vi "Agilent B2900 Series Output DC Volts.vi"() -> ()   [LabVIEW 2023]
doc: "This example shows how to configure the instrument's output voltage level, over current protection, and over voltage protection. The actual voltage level and actual current level are returned as well as whether over voltage protection (OVP) or over current protection (OCP) has been tripped."
uses:
  Agilent B2900 Series.lvlib
panel:
  in  "Source Range (V)":dbl=2.0
  in  "Voltage Level (V)":dbl
  in  "Compliance Current (0.0001 A)":dbl=0.0001
  in  "Enable Output Protection (T: Enable)":bool=TRUE
  in  "Stop Output":bool
  out "OCP Tripped?":bool
  out "Actual Current Level (A)":dbl format="%_6g"
  out "Actual Voltage Level (V)":dbl format="%_6g"
  in  "Channel (0: Channel 1)":i32(ring) items=["Channel 1", "Channel 2"]
  in  "VISA resource name":refnum<visa-resource-name>
  # "(c) 2011-2021 National Instruments.  ALL RIGHTS RESERVED."
  # "Compliance Protection"
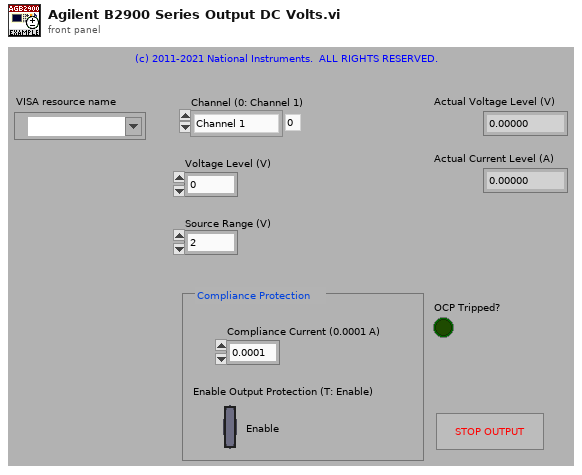
[diagram p1: front panel]
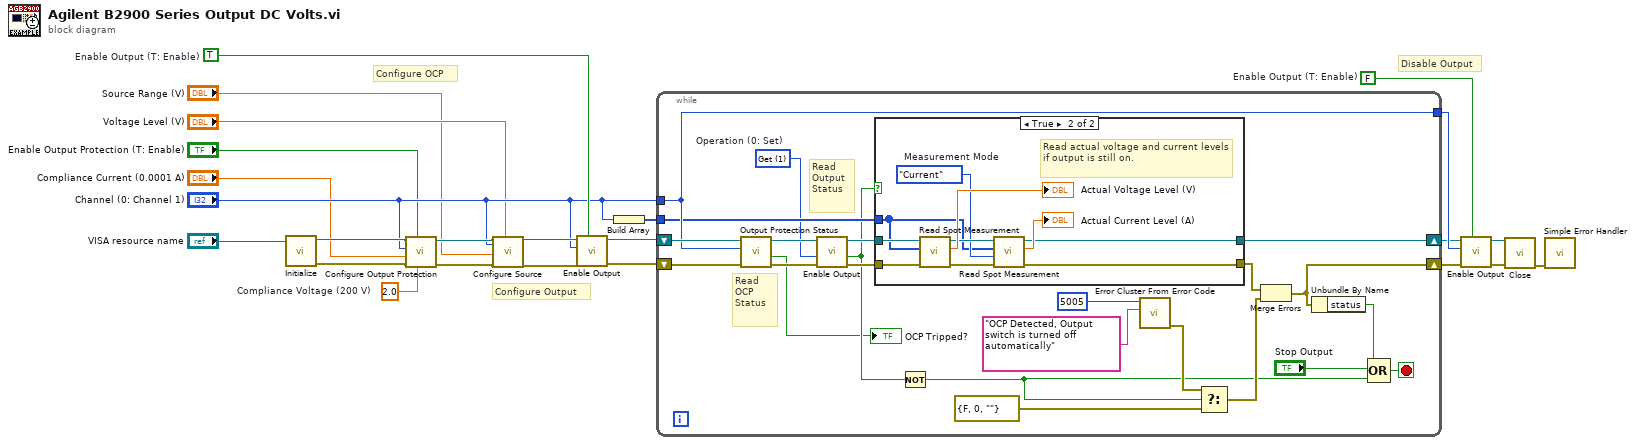
[diagram p0: block diagram]
diagram:
  w4 = 2.0  # Compliance Voltage (200 V)
  w15 = FALSE  # Enable Output (T: Enable)
  w14 = TRUE  # Enable Output (T: Enable)
  # "Disable Output"
  # "Configure Output"
  # "Configure OCP"
  n1 = call "Initialize.vi"("VISA resource name"="VISA resource name") -> ("error out"=w11:errorcluster, "VISA resource name out"=w12:refnum<visa-resource-name>)  [unwired: 9 in]
  n2 = call "Configure Output Protection.vi"("Compliance Voltage (2 V)"=w4, "Enable Output Protection (T: Enable)"="Enable Output Protection (T: Enable)", "error in (no error)"=w11, "Compliance Current (0.0001 A)"="Compliance Current (0.0001 A)", "Channel (0: Channel 1)"="Channel (0: Channel 1)", "VISA resource name"=w12) -> ("error out"=w9:errorcluster, "VISA resource name out"=w10:refnum<visa-resource-name>)  [unwired: 4 in]
  n3 = call "Configure Source.vi"("VISA resource name"=w10, "Channel (0: Channel 1)"="Channel (0: Channel 1)", "Source Range (2)"="Source Range (V)", "error in (no error)"=w9, "Output Level (0)"="Voltage Level (V)") -> ("VISA resource name out"=w8:refnum<visa-resource-name>, "error out"=w7:errorcluster)  [unwired: 13 in]
  n4 = call "Enable Output.vi"("Enable Output (F: Disable)"=w14, "error in (no error)"=w7, "Channel (0: Channel 1)"="Channel (0: Channel 1)", "VISA resource name"=w8) -> ("error out"=w21:errorcluster, "VISA resource name out"=w22:refnum<visa-resource-name>)  [unwired: 5 in, 1 out]
  n5 = Build Array("Channel (0: Channel 1)") -> (w13:i32[])
  n6 = while {
    tunnel: "Channel (0: Channel 1)" -> [w45]
    tunnel: [w45] -> w20
    shift-right: [w33] -> w19
    shift-left: w21 -> [w46]
    tunnel: w13 -> [w43]
    shift-right: [w44] -> w16
    shift-left: w22 -> [w47]
    stop <- w40 stop-if-true
    w31 = 1 items=["Set", "Get"]  # Operation (0: Set)
    # "Read Output Status"
    # "Read OCP Status"
    n7 = call "Output Protection Status.vi"("error in (no error)"=w46, "Channel (0: Channel 1)"=w45, "VISA resource name"=w47) -> ("error out"=w30:errorcluster, "OCP Tripped?"=→"OCP Tripped?":bool, "VISA resource name out"=w32:refnum<visa-resource-name>)  [unwired: 5 in, 1 out]
    n8 = call "Enable Output.vi"("error in (no error)"=w30, "Operation (0: Set)"=w31, "VISA resource name"=w32) -> ("error out"=w29:errorcluster, "Output Enabled?"=w27:bool, "VISA resource name out"=w28:refnum<visa-resource-name>)  [unwired: 6 in]
    n9 = case shown="True" w27 {
      tunnel: w28 -> [w49 w59]
      tunnel: w29 -> [w48 w58]
      tunnel: [w48 w50] -> w34
      tunnel: [w49 w52] -> w44
      tunnel: w43 -> [_ w51]
      frame False {
        # "Stop measurement if output is turned off."
      }
      frame True {
        w54 = enum16{"Voltage", "Current", "Resistance"}."Current"  # Measurement Mode
        # "Read actual voltage and current levels if output is still on."
        n10 = call "Read Spot Measurement.vi"("error in (no error)"=w58, "Channel List ({Channel1})"=w51, "VISA resource name"=w59) -> ("error out"=w57:errorcluster, "Measurement Result"=→"Actual Voltage Level (V)":dbl, "VISA resource name out"=w55:refnum<visa-resource-name>)  [unwired: 6 in]
        n11 = call "Read Spot Measurement.vi"("error in (no error)"=w57, "Measurement Mode (0:Voltage)"=w54, "Channel List ({Channel1})"=w51, "VISA resource name"=w55) -> ("error out"=w50:errorcluster, "Measurement Result"=→"Actual Current Level (A)":dbl, "VISA resource name out"=w52:refnum<visa-resource-name>)  [unwired: 5 in]
      }
    }
    n12 = Not(x=w27) -> (.not. x?=w26:bool)
    n13 = call <vilib>:"Error Cluster From Error Code.vi"("error message (\"\")"="OCP Detected, Output switch is turned off automatically" ("error message (\"\")"), "error code (0)"=5005) -> ("error out"=w37:errorcluster)  [unwired: 7 in]
    n14 = Select(t=w37, s=w26, f=errorcluster {"status"=FALSE, "code"=0, "source"=""} ("error in 3 (no error)")) -> (s? t:f=w36:errorcluster)
    n15 = Merge Errors(w34, w36) -> (w33:errorcluster)
    n16 = Unbundle By Name(w33) -> ("status"=w42:bool)
    n17 = Compound Arithmetic op=OR(w42, "Stop Output", w26) -> (w40:bool)
  }
  n18 = call "Enable Output.vi"("Enable Output (F: Disable)"=w15, "error in (no error)"=w19, "Channel (0: Channel 1)"=w20, "VISA resource name"=w16) -> ("error out"=w17:errorcluster, "VISA resource name out"=w18:refnum<visa-resource-name>)  [unwired: 5 in, 1 out]
  n19 = call "Close.vi"("error in (no error)"=w17, "VISA resource name"=w18) -> ("error out"=w23:errorcluster)  [unwired: 9 in]
  n20 = call <vilib>:"Simple Error Handler.vi"("error in (no error)"=w23) -> ()  [unwired: 4 in, 5 out]
